vi "send mirror shape.vi"(8 "error in (no error)":errorcluster, 11 "RSA in":refnum<class "RSA.lvclass">) -> (0 "error out":errorcluster, 3 "RSA out":refnum<class "RSA.lvclass">)   [LabVIEW 2012, in "RSA.lvclass"]
uses:
  RSA.lvclass
  RSA.lvclass/RSA.ctl
  <vilib>/Distrio/Murmex/Murmex/Murmex.lvclass
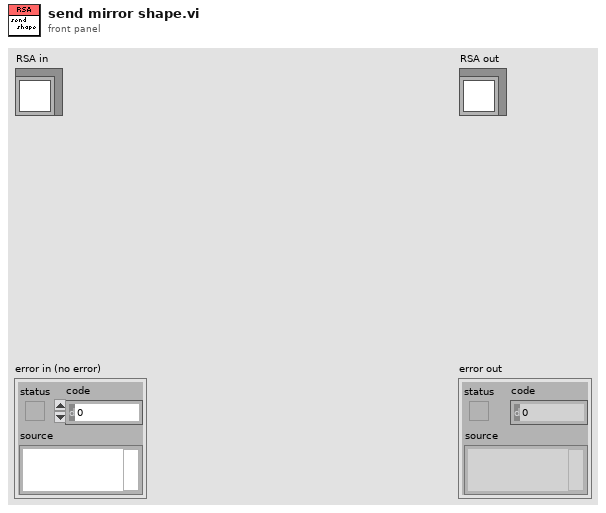
[diagram p1: front panel]
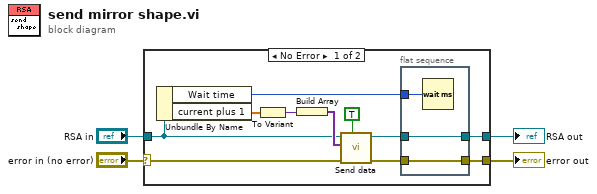
[diagram p0: block diagram]
diagram:
  n1 = case shown="No Error" "error in (no error)" {
    selector: "error in (no error)" -> [w12 w20]
    tunnel: [w5 w20] -> w3
    tunnel: [w7 w19] -> w1
    tunnel: "RSA in" -> [w11 w19]
    frame No Error {
      n2 = Unbundle By Name(w11) -> ("Wait time"=w9:u32, "current plus 1"=w10:dbl[])
      n3 = To Variant(anything=w10) -> (Variant=w13:variant)
      n4 = Build Array(w13) -> (w14:variant[])
      n5 = call <vilib>:"Send data.vi"("is finalised data? (T)"=TRUE, "error in (no error)"=w12, "data (channels array)"=w14, "Murmex in"=w11) -> ("error out"=w6:errorcluster, "Murmex out"=w8:refnum<class "RSA.lvclass">)  [unwired: 6 in]
      n6 = flat-sequence {
        tunnel: w9 -> [w18]
        tunnel: w8 -> [w17]
        tunnel: [w17] -> w7
        tunnel: w6 -> [w16]
        tunnel: [w16] -> w5
        frame #0 {
          n7 = Wait (ms)(milliseconds to wait=w18) -> ()  [unwired: 1 out]
        }
      }
    }
    frame Error {
    }
  }
  "error out" <- w3
  "RSA out" <- w1
